vi "Zip and delete folder.vi"(1 "Delete folder after zipping?":bool, 2 "Directory to zip":path) -> (0 "Error Out":errorcluster)   [LabVIEW 2015]
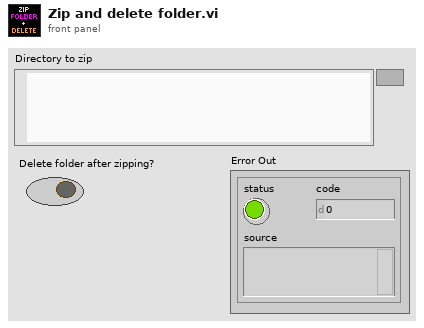
[diagram p1: front panel]
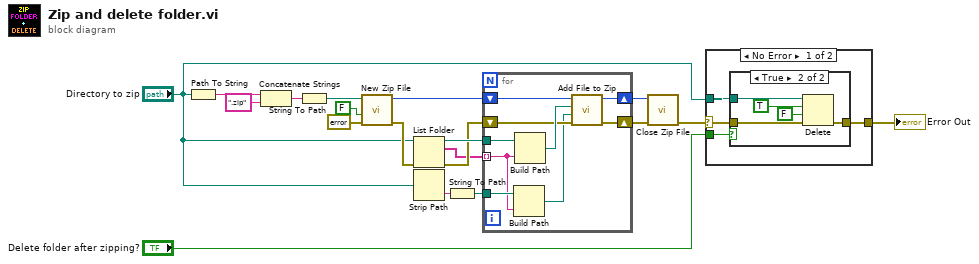
[diagram p0: block diagram]
diagram:
  n1 = Path To String(path="Directory to zip") -> (string=w9:string)
  n2 = Concatenate Strings(w9, ".zip" ("string")) -> (w8:string)
  n3 = String To Path(string=w8) -> (path=w7:path)
  n4 = call <vilib>:"New Zip File.vi"("error in (no error)"=errorcluster {"status"=FALSE, "code"=0, "source"=""}, "confirm overwrite? (F)"=FALSE, "target"=w7) -> ("error out"=w13:errorcluster, "zip file out"=w18:i64)  [unwired: 2 in, 1 out]
  n5 = List Folder(path="Directory to zip", error in=w13) -> (path out=w12:path, filenames=w10:string[], error out=w11:errorcluster)  [unwired: 2 in, 1 out]
  n6 = Strip Path(path="Directory to zip") -> (name=w2:string)  [unwired: 1 out]
  n7 = String To Path(string=w2) -> (path=w1:path)
  n8 = for {
    tunnel: w12 -> [w24]
    shift-right: [w27] -> w17
    shift-left: w18 -> [w28]
    shift-right: [w26] -> w16
    shift-left: w11 -> [w23]
    tunnel: w10 -> [w21] mode=indexing
    tunnel: w1 -> [w22]
    n9 = Build Path(base path=w22, name or relative path=w21) -> (appended path=w20:path)
    n10 = Build Path(base path=w24, name or relative path=w21) -> (appended path=w25:path)
    n11 = call <vilib>:"Add File to Zip.vi"("error in (no error)"=w23, "destination path in zip"=w20, "source file path"=w25, "zip file in"=w28) -> ("error out"=w26:errorcluster, "zip file out"=w27:i64)  [unwired: 6 in]
  }
  n12 = call <vilib>:"Close Zip File.vi"("error in (no error)"=w16, "zip file in"=w17) -> ("error out"=w6:errorcluster)  [unwired: 5 in]
  n13 = case shown="No Error" w6 {
    selector: w6 -> [w31 w39]
    tunnel: "Delete folder after zipping?" -> [w32 _]
    tunnel: [w30 w39] -> w4
    tunnel: "Directory to zip" -> [w29 _]
    frame No Error {
      n14 = case shown="True" w32 {
        tunnel: w31 -> [w33 w37]
        tunnel: [w33 w36] -> w30
        tunnel: w29 -> [_ w34]
        frame False {
        }
        frame True {
          n15 = Delete(path (use dialog)=w34, entire hierarchy (F)=TRUE, confirm (F)=FALSE, error in=w37) -> (error out=w36:errorcluster)  [unwired: 1 in, 2 out]
        }
      }
    }
    frame Error {
    }
  }
  "Error Out" <- w4
